vi "fgv_error.vi"(7 "cmd":T2, 8 "error in (no error)":errorcluster, 11 "error cluster":T1) -> (0 "error out":errorcluster, 3 "error cluster 2":T1)   [LabVIEW 2019]
uses:
  _ctrl/rw.ctl
  _ctrl/Error list.ctl
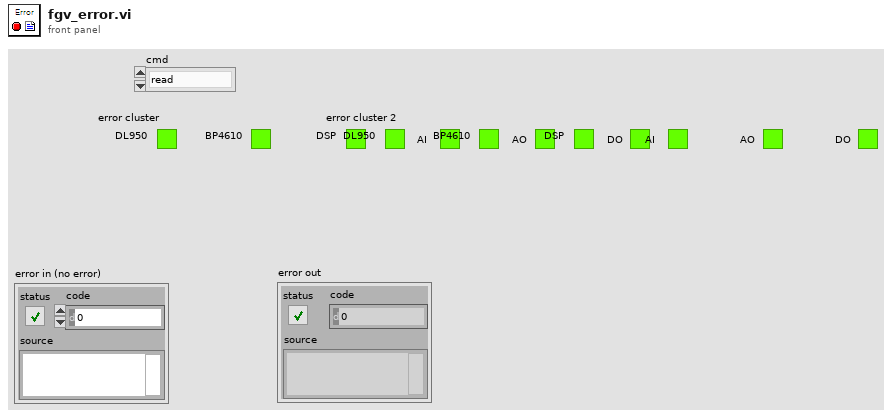
[diagram p1: front panel]
types:
  T1 = typedef "Error list.ctl" = cluster{"DL950":bool, "BP4610":bool, "DSP":bool, "AI":bool, "AO":bool, "DO":bool}
  T2 = typedef "rw.ctl" = enum16{"read", "write"}
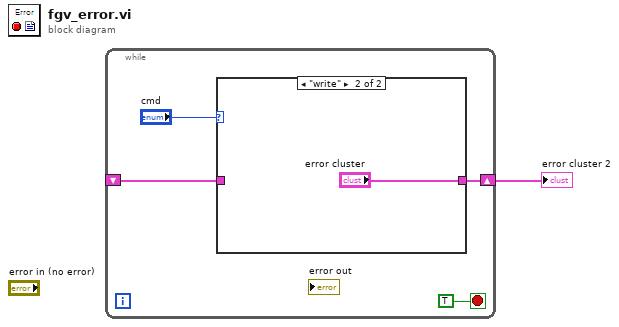
[diagram p0: block diagram]
diagram:
  n1 = while {
    shift-right: [w3] -> w1
    shift-left: _ -> [w2]
    stop <- TRUE stop-if-true
    n2 = case shown="\"write\"" "cmd" {
      tunnel: [w6 "error cluster"] -> w3
      tunnel: w2 -> [w6 _]
      frame "read", Default {
      }
      frame "write" {
      }
    }
  }
  "error cluster 2" <- w1
